vi "Camera Identification Helper.vi"() -> ()   [LabVIEW 2011]
uses:
  <vilib>/vision/driver/NI_Vision_Acquisition_Software.lvlib
panel:
  out "Image":T1(plugin-control)
  out "Camera Info":T2 {"SerialNumberHigh" format="%x"; "SerialNumberLow" format="%x"}
  in  "camera number":i32
  in  "stop":bool
  out "error out":errorcluster
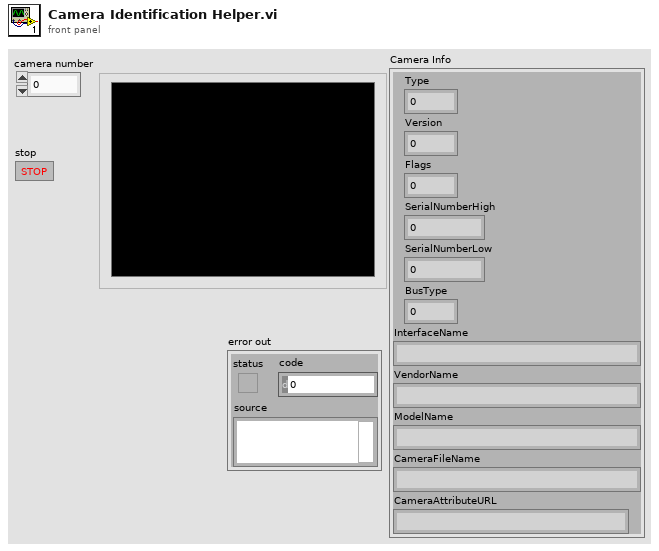
[diagram p1: front panel]
types:
  T1 = typedef "IMAQ Image.ctl" = refnum<image>
  T2 = cluster{"Type":u32, "Version":u32, "Flags":u32, "SerialNumberHigh":u32, "SerialNumberLow":u32, "BusType":u32, "InterfaceName":string, "VendorName":string, "ModelName":string, "CameraFileName":string, "CameraAttributeURL":string}
  T3 = cluster{"Type":u32, "Version":u32, "Flags":u32, "SerialNumberHigh":u32, "SerialNumberLow":u32, "BusType":u32, "InterfaceName":string, "VendorName":string, "ModelName":string, "CameraFileName":string, "CameraAttributeURL":string}[]
  T4 = typedef "IMAQdx.ctl" = refnum<k21>
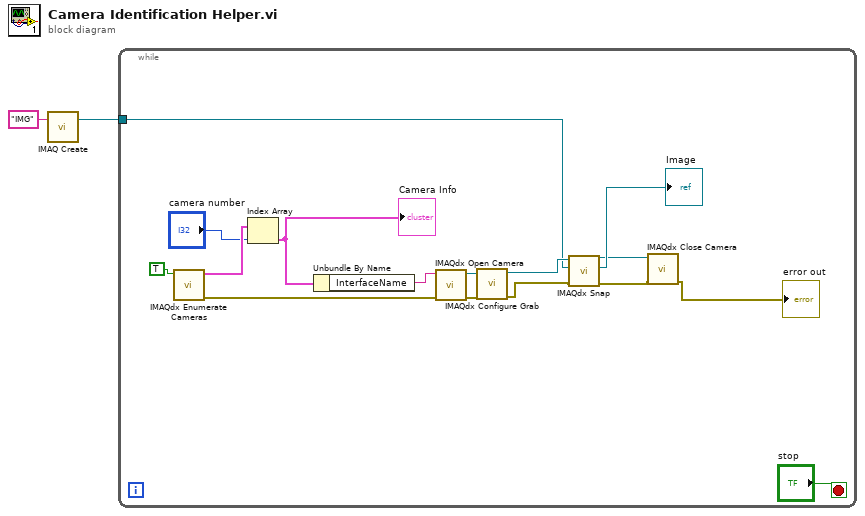
[diagram p0: block diagram]
diagram:
  n1 = call "IMAQ Create"("Image Name"="IMG") -> ("New Image"=w1:T1)  [unwired: 4 in, 1 out]
  n2 = while {
    tunnel: w1 -> [w7]
    stop <- "stop" stop-if-true
    n3 = call <vilib>:"IMAQdx Enumerate Cameras.vi"("Connected Only? (Yes)"=TRUE) -> ("error out"=w17:errorcluster, "Camera Information Array"=w12:T3)  [unwired: 9 in]
    n4 = Index Array(array=w12, index="camera number") -> (element=w11:T2)
    "Camera Info" <- w11
    n5 = Unbundle By Name(w11) -> ("InterfaceName"=w16:string)
    n6 = call <vilib>:"IMAQdx Open Camera.vi"("error in"=w17, "Session In"=w16) -> ("error out"=w14:errorcluster, "Session Out"=w15:T4)  [unwired: 8 in]
    n7 = call <vilib>:"IMAQdx Configure Grab.vi"("error in"=w14, "Session In"=w15) -> ("error out"=w8:errorcluster, "Session Out"=w9:T4)  [unwired: 8 in]
    n8 = call <vilib>:"IMAQdx Snap.vi"("error in"=w8, "Image In"=w7, "Session In"=w9) -> ("error out"=w4:errorcluster, "Image Out"=→"Image":T1, "Session Out"=w5:T4)  [unwired: 6 in]
    n9 = call <vilib>:"IMAQdx Close Camera.vi"("error in"=w4, "Session In"=w5) -> ("error out"=→"error out":errorcluster)  [unwired: 9 in]
  }
